vi "tcp_get_mode.vi"(7 "button_get_mode":bool, 8 "error in":errorcluster, 9 "tcp_connected_in":bool, 10 "new_connection_in":bool, 11 "connection_id_in":refnum<k5>) -> (0 "error out":errorcluster, 1 "tcp_connected_out":bool, 2 "new_data_available":bool, 3 "connection_id_out":refnum<k5>, 6 "data_out":T1)   [LabVIEW 2025]
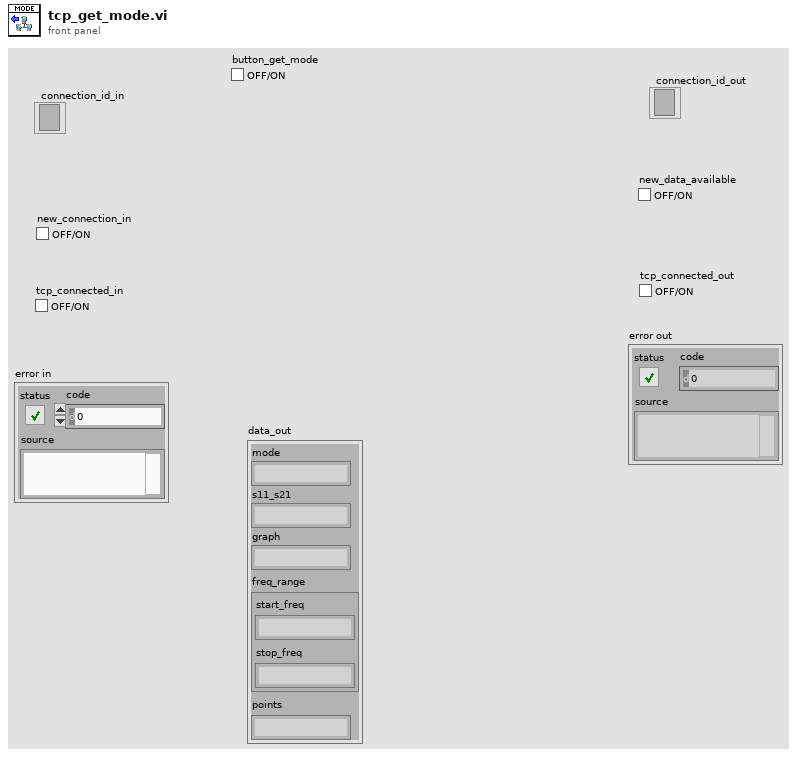
[diagram p1: front panel]
types:
  T1 = cluster{"mode":string, "s11_s21":string, "graph":string, "freq_range":cluster{"start_freq":string, "stop_freq":string}, "points":string}
  T2 = cluster{"result string":string, "result string":string}
  T3 = cluster{string, "result string":string, "result string":string, cluster{"result string":string, "result string":string}, "result string":string}
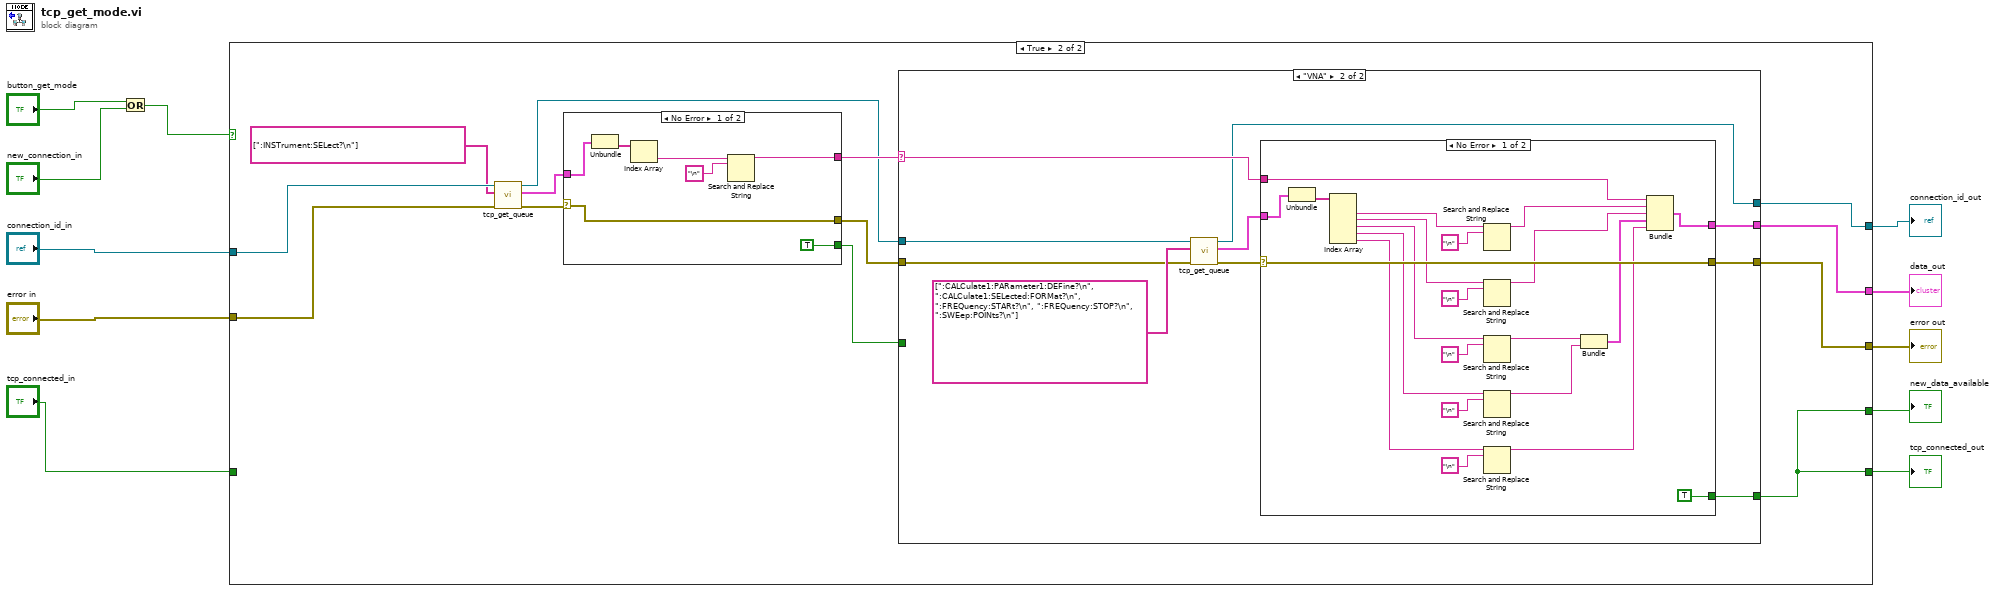
[diagram p0: block diagram]
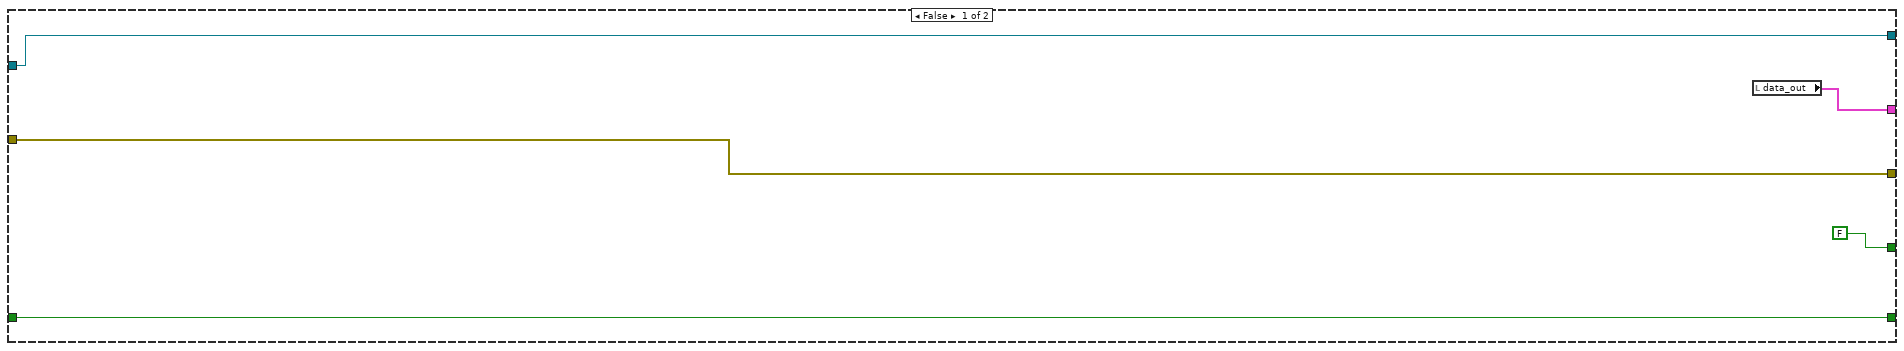
[diagram p2: hidden frame]
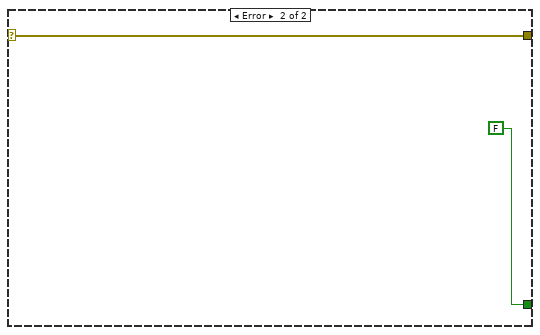
[diagram p4: hidden frame]
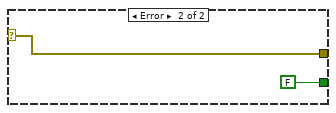
[diagram p5: hidden frame]
diagram:
  n1 = Or(x="button_get_mode", y="new_connection_in") -> (x .or. y?=w3:bool)
  n2 = case shown="True" w3 {
    tunnel: [w15 w21] -> w10
    tunnel: [w16 w19] -> w9
    tunnel: "connection_id_in" -> [w16 w27]
    tunnel: "error in" -> [w15 w26]
    tunnel: [FALSE ("tcp_connected_in") w17] -> w5
    tunnel: [w13 w22] -> w4
    tunnel: [w12 w17] -> w2
    tunnel: "tcp_connected_in" -> [w12 _]
    frame False {
      n3 = local read "data_out"() -> (w13:T1)
    }
    frame True {
      n4 = call "tcp_get_queue.vi"("error in"=w26, "command queue"=string[] [":INSTrument:SELect?\n"], "connection in"=w27) -> ("error out"=w29:errorcluster, "output"=w28:cluster{string[], string[]}, "connection out"=w20:refnum<k5>)  [unwired: 6 in]
      n5 = case shown="No Error" w29 {
        selector: w29 -> [w71 w75]
        tunnel: w28 -> [w73 _]
        tunnel: [w71 w75] -> w23
        tunnel: [w68 _] -> w24
        tunnel: [TRUE FALSE] -> w18
        frame No Error {
          n6 = Unbundle(w73) -> (w72:string[])  [unwired: 1 out]
          n7 = Index Array(array=w72) -> (element=w69:string)  [unwired: 1 in]
          n8 = Search and Replace String(input string=w69, search string="\n") -> (result string=w68:string)  [unwired: 6 in, 3 out]
        }
        frame Error {
        }
      }
      n9 = case shown="\"VNA\"" w24 {
        selector: w24 -> [_ w38]
        tunnel: w23 -> [w32 w41]
        tunnel: [_ w37] -> w22
        tunnel: [w30 w36] -> w17
        tunnel: [w32 w35] -> w21
        tunnel: w20 -> [w31 w34]
        tunnel: [w31 w33] -> w19
        tunnel: w18 -> [w30 _]
        frame "SA", Default {
        }
        frame "VNA" {
          n10 = call "tcp_get_queue.vi"("error in"=w41, "command queue"=string[] [":CALCulate1:PARameter1:DEFine?\n", ":CALCulate1:SELected:FORMat?\n", ":FREQuency:STARt?\n", ":FREQuency:STOP?\n", ":SWEep:POINts?\n"], "connection in"=w34) -> ("error out"=w39:errorcluster, "output"=w40:cluster{string[], string[]}, "connection out"=w33:refnum<k5>)  [unwired: 6 in]
          n11 = case shown="No Error" w39 {
            selector: w39 -> [w60 w65]
            tunnel: w40 -> [w64 _]
            tunnel: [w62 _] -> w37
            tunnel: [TRUE FALSE] -> w36
            tunnel: [w60 w65] -> w35
            tunnel: w38 -> [w53 _]
            frame No Error {
              n12 = Unbundle(w64) -> (w63:string[])  [unwired: 1 out]
              n13 = Index Array(array=w63) -> (element #1=w58:string, element #2=w55:string, element #3=w50:string, element #4=w49:string, element #5=w44:string)  [unwired: 5 in]
              n14 = Search and Replace String(input string=w58, search string="\n") -> (result string=w57:string)  [unwired: 6 in, 3 out]
              n15 = Search and Replace String(input string=w55, search string="\n") -> (result string=w54:string)  [unwired: 6 in, 3 out]
              n16 = Search and Replace String(input string=w50, search string="\n") -> (result string=w48:string)  [unwired: 6 in, 3 out]
              n17 = Search and Replace String(input string=w49, search string="\n") -> (result string=w47:string)  [unwired: 6 in, 3 out]
              n18 = Search and Replace String(input string=w44, search string="\n") -> (result string=w43:string)  [unwired: 6 in, 3 out]
              n19 = Bundle("result string"=w48, "result string"=w47) -> (w46:T2)  [unwired: 1 in]
              n20 = Bundle(w53, "result string"=w57, "result string"=w54, w46, "result string"=w43) -> (w62:T3)  [unwired: 1 in]
            }
            frame Error {
            }
          }
        }
      }
    }
  }
  "error out" <- w10
  "tcp_connected_out" <- w2
  "connection_id_out" <- w9
  "new_data_available" <- w5
  "data_out" <- w4
